vi "FakeImageSignalGenerator.vi"(8 "Z":dbl, 9 "Y":dbl=1.0, 10 "X":dbl) -> (2 "E":dbl)   [LabVIEW 2014, in "GenericDAQ.lvlib"]
doc: "This template is the starting point for creating a model function to be passed to the Nonlinear Curve Fit.vi."
uses:
  <instrlib>/GenericDAQ/GenericDAQ.lvlib
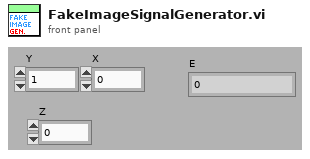
[diagram p1: front panel]
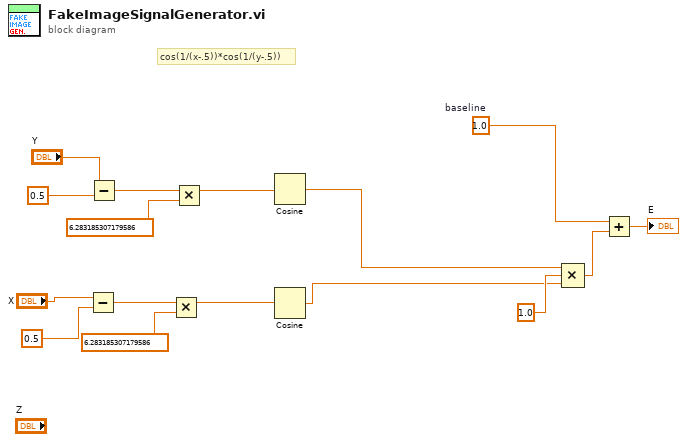
[diagram p0: block diagram]
diagram:
  w14 = 1.0  # baseline
  # "cos(1/(x-.5))*cos(1/(y-.5))"
  n1 = Subtract(x="X", y=0.5 ("focus_pos")) -> (x-y=w7:dbl)
  n2 = Subtract(x="Y", y=0.5 ("focal plane pos")) -> (x-y=w8:dbl)
  n3 = Multiply(x=w7, y=6.283185307179586) -> (x*y=w4:dbl)
  n4 = Multiply(x=w8, y=6.283185307179586) -> (x*y=w3:dbl)
  n5 = Cosine(x=w3) -> (cos(x)=w6:dbl)
  n6 = Cosine(x=w4) -> (cos(x)=w5:dbl)
  n7 = Compound Arithmetic op=MULTIPLY(w6, 1.0 ("value"), w5) -> (w16:dbl)
  n8 = Add(x=w14, y=w16) -> (x+y=→"E":dbl)
